vi "CreateRxSession.vi"(8 "error in (no error)":errorcluster, 11 "NI-XNET in":refnum<class "NI-XNET.lvclass">) -> (0 "error out":errorcluster, 3 "NI-XNET out":refnum<class "NI-XNET.lvclass">)   [LabVIEW 2023, in "HardwareAbstractionLayer_LVOOP.lvlib" / "CAN HAL Lib.lvlib" / "NI-XNET.lvclass"]
uses:
  NI-XNET.lvclass
  NI-XNET.lvclass/NI-XNET.ctl
  <vilib>/xnet/xnet.llb/XNET Create Session (Frame Input Stream).vi
  <resource>/objmgr/xnet.rc
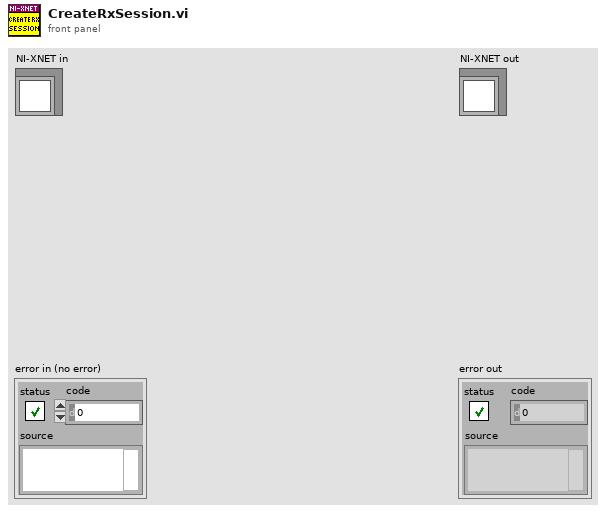
[diagram p1: front panel]
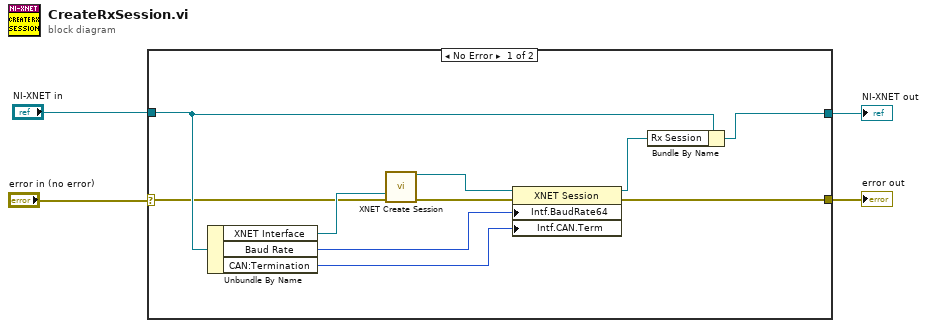
[diagram p0: block diagram]
diagram:
  n1 = case shown="No Error" "error in (no error)" {
    selector: "error in (no error)" -> [w5 w15]
    tunnel: "NI-XNET in" -> [w9 w16]
    tunnel: [w7 w16] -> w2
    tunnel: [w6 w15] -> w1
    frame No Error {
      n2 = Unbundle By Name(w9) -> ("XNET Interface"=w12:refnum<k21>, "Baud Rate"=w11:u64, "CAN:Termination"=w10:u32)
      n3 = call-poly <vilib>:"XNET Create Session.vi"("interface"=w12, "error in (no error)"=w5) -> ("session out"=w14:refnum<k21>, "error out"=w13:errorcluster)  [unwired: 12 in]
      n4 = property class="XNET Session"(reference=w14, error in=w13, "Intf.BaudRate64"=w11, "Intf.CAN.Term"=w10) -> (reference out=w8:refnum<k21>, error out=w6:errorcluster)
      n5 = Bundle By Name(cluster=w9, "Rx Session"=w8) -> (w7:refnum<class "NI-XNET.lvclass">)
    }
    frame Error {
    }
  }
  "error out" <- w1
  "NI-XNET out" <- w2
